vi "closeEngine.vi"(8 "error in (no error)":errorcluster, 11 "Simon_Engine in":refnum<class "Simon_Engine.lvclass">) -> (0 "error out":errorcluster, 3 "Simon_Engine out":refnum<class "Simon_Engine.lvclass">)   [LabVIEW 2020, in "Simon_Engine.lvclass"]
uses:
  Simon_Engine.lvclass
  Simon_Engine.lvclass/Simon_Engine.ctl
  LED/LED Class/LED.lvclass
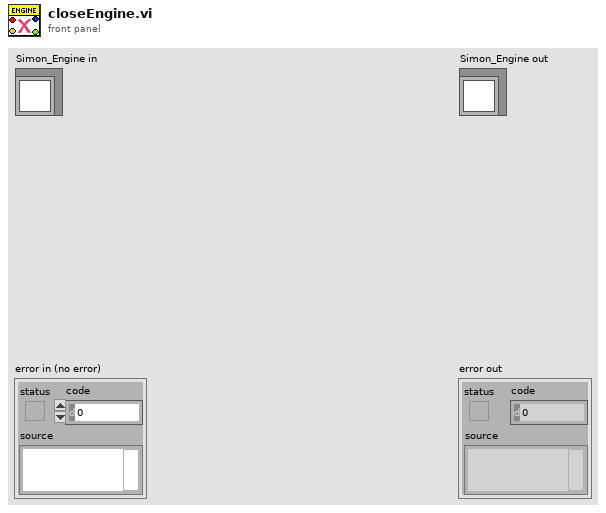
[diagram p1: front panel]
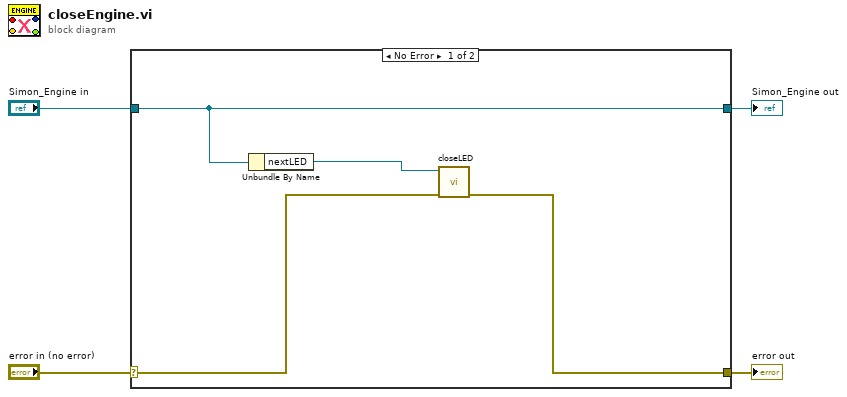
[diagram p0: block diagram]
diagram:
  n1 = case shown="No Error" "error in (no error)" {
    selector: "error in (no error)" -> [w6 w10]
    tunnel: [w5 w10] -> w3
    tunnel: [w8 w9] -> w1
    tunnel: "Simon_Engine in" -> [w8 w9]
    frame No Error {
      n2 = Unbundle By Name(w8) -> ("nextLED"=w7:refnum<class "LED.lvclass">)
      n3 = call "closeLED.vi"("error in (no error)"=w6, "LED in"=w7) -> ("error out"=w5:errorcluster)  [unwired: 9 in]
    }
    frame Error {
    }
  }
  "error out" <- w3
  "Simon_Engine out" <- w1
